vi "Logger.PGSQL.WriteVariableMultiline.vi"(6 "Timestamps":timestamp[](array[timestamp]), 8 "error in (no error)":errorcluster, 9 "Data":variant, 10 "Address":string, 11 "Logger":refnum<class "Logger.PGSQL.lvclass">) -> (0 "error out":errorcluster, 3 "Logger out":refnum<class "Logger.PGSQL.lvclass">)   [LabVIEW 2019, in "Logger.PGSQL.lvlib" / "Logger.PGSQL.lvclass"]
doc: "<b>Address</b> list of database addresses, seprated by new lines\n<b>Data</b> Array of clusters, where each cluster element corresponds to an address\n<b>Timestamps</b> Array of timestamps correspoding to each element of Data array\n\n---------------------------------------------------------------\nJKI State Machine Objects™\nhttp://jki.net/state-machine-objects/\nCopyright (C) 2005-2015, JKI <info@jki.net>\nALL RIGHTS RESERVEDJKI State Machine Objects (SMO) 1.0.0.4\nJKI - JKI\nCopyright (c) 2015, JKI"
uses:
  Logger.PGSQL.lvclass
  Typedefs/PrivateEvents--Logger.PGSQL.Write Variable Multiline.ctl
panel:
  # "For instructions on how to use the JKI State Machine Objects, examples and video tutorials, visit:\nhttp://jki.net/state-machine-objects/\n\nJKI State Machine Objects™\nhttp://jki.net/state-machine-objects/\nCopyright (C) 2005-2015, JKI <info@jki.net>\nALL RIGHTS RESERVED"
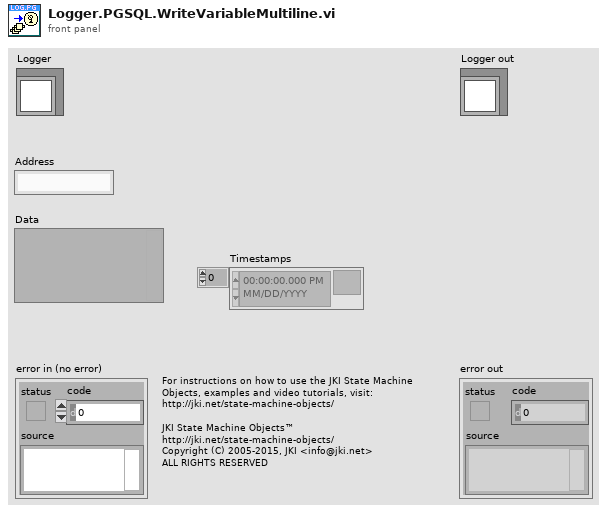
[diagram p1: front panel]
types:
  T1 = typedef "Logger.PGSQL.lvlib/Logger.PGSQL.lvclass/PrivateEvents--Logger.PGSQL.Write Variable Multiline.ctl" = cluster{"Address":string, "Data":variant, "Timestamps":timestamp[]}
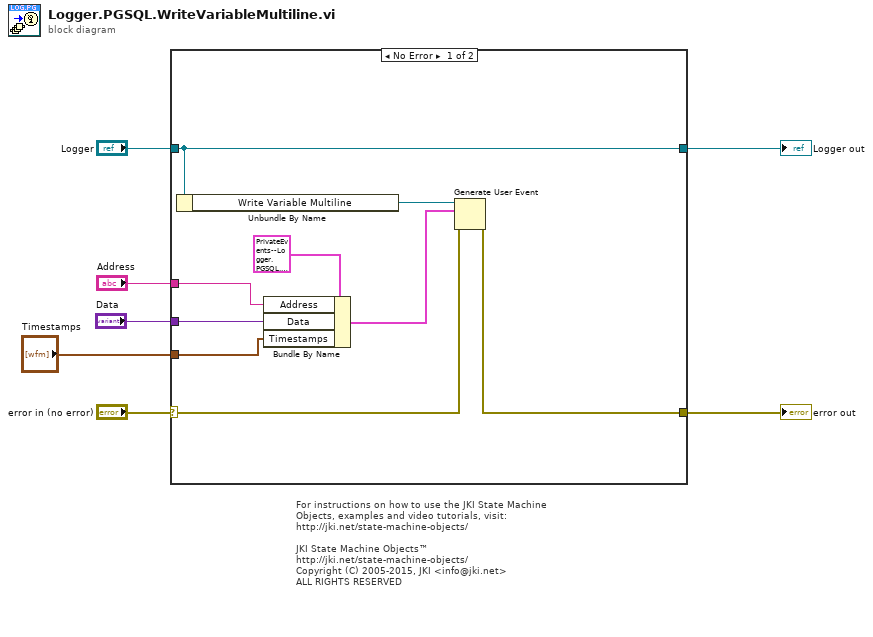
[diagram p0: block diagram]
diagram:
  # "For instructions on how to use the JKI State Machine Objects, examples and video tutorials, visit:\nhttp://jki.net/state-machine-objects/\n\nJKI State Machine Objects™\nhttp://jki.net/state-machine-objects/\nCopyright (C) 2005-2015, JKI <info@jki.net>\nALL RIGHTS RESERVED"
  n1 = case shown="No Error" "error in (no error)" {
    selector: "error in (no error)" -> [w16 w18]
    tunnel: [w14 w18] -> w6
    tunnel: [w13 w17] -> w7
    tunnel: "Logger" -> [w13 w17]
    tunnel: "Address" -> [w12 _]
    tunnel: "Data" -> [w11 _]
    tunnel: "Timestamps" -> [w8 _]
    frame No Error {
      n2 = Unbundle By Name(w13) -> ("Write Variable Multiline"=w15:refnum<user-event>)
      n3 = Bundle By Name(cluster=T1 {"Address"="", "Data"=variant, "Timestamps"=[]} ("Write Variable"), "Address"=w12, "Data"=w11, "Timestamps"=w8) -> (w10:T1)
      n4 = Generate User Event(user event=w15, event data cluster=w10, error in=w16) -> (error out=w14:errorcluster)  [unwired: 1 in, 1 out]
    }
    frame Error {
    }
  }
  "error out" <- w6
  "Logger out" <- w7
